vi "Fpga_v5.vi"() -> ()   [LabVIEW 2015]
uses:
  <vilib>/rvi/Emulation/niFpgaGetClockAttributes.vi
  <vilib>/rvi/Emulation/niFpgaSctlEmulationGetInTimedLoop.vi
  <vilib>/rvi/Emulation/niFpgaEmulationReportErrorSimple.vi
  <vilib>/rvi/eio/common/nirviEmuTemplateMethod_errors.vi
  <vilib>/rvi/Emulation/niFpgaCriticalErrorInLSC.vi
  <vilib>/rvi/interface/RandomDataEmulation/niFpgaRandomDataHandleErrors.vi
  <vilib>/eio/EIONode/EIONode.xnode
  <vilib>/rvi/DataTransferAndStorage/Container/XNode/niFpgaContainer.xnode
  <vilib>/rvi/interface/RandomDataEmulation/nirviRandomDataFpgaReadWriteTemplate.vi
panel:
  out "x-y 4":u32
  out "Mod2/DIO6_B 2":bool
  out "x-y":u32
  in  "Data write ON/OFF":bool
  out "Mod2/DIO6_B":bool
  out "Timed Out?":bool
  out "x-y 3":u32
  in  "stop":bool
  in  "Mod4/AO0 2":i16
  out "Mod3/AI0 2":fxp<+/-,16,5>
  out "Boolean 2":bool
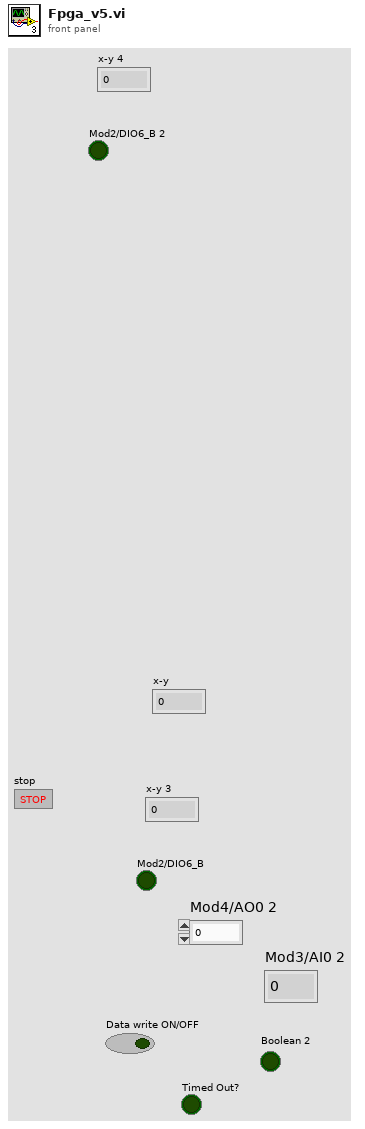
[diagram p1: front panel]
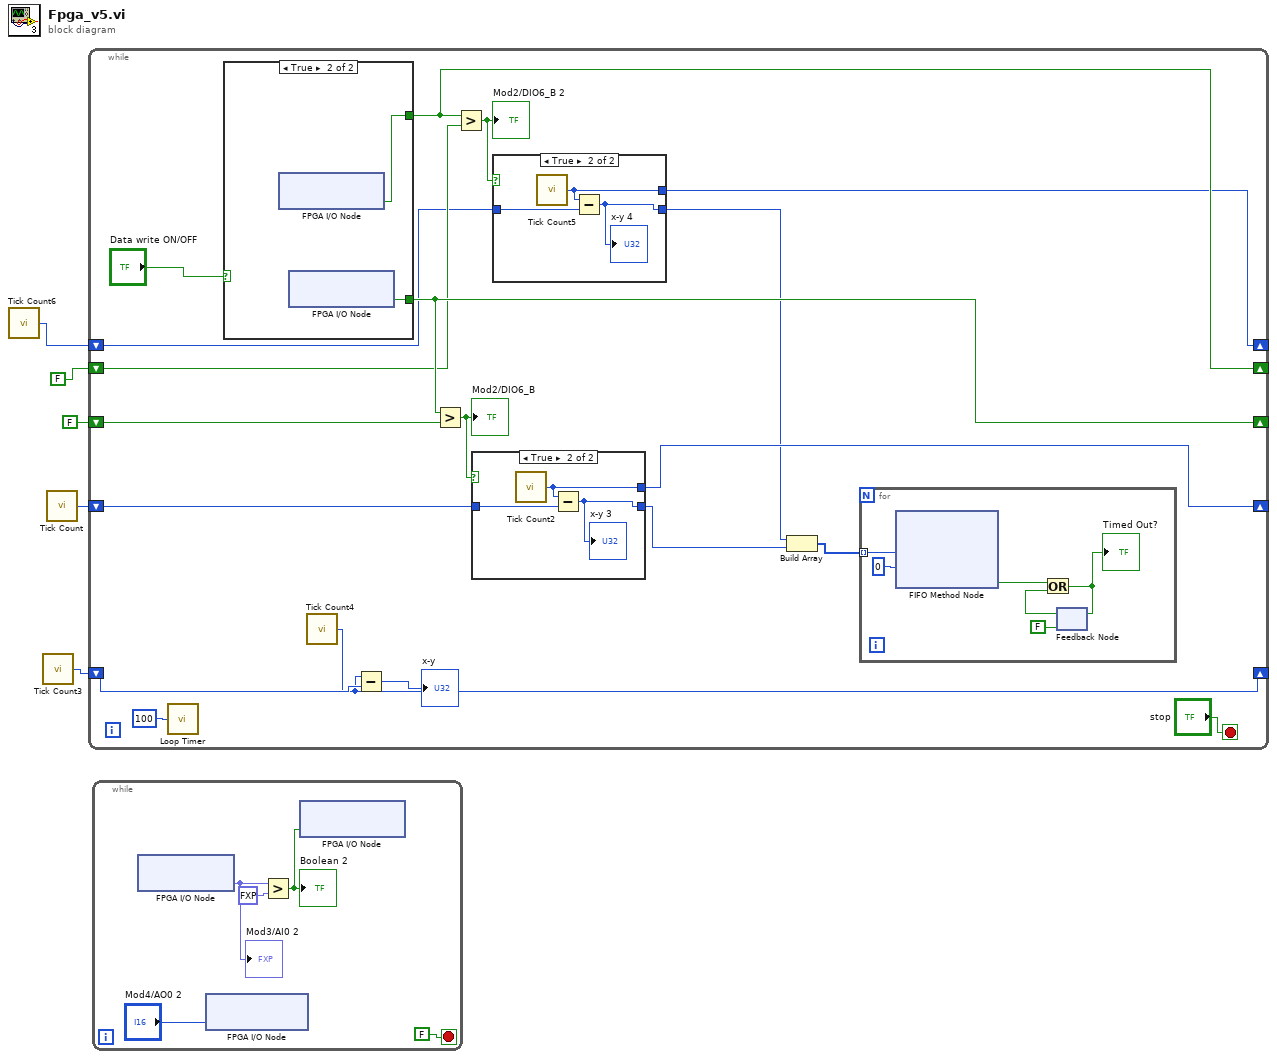
[diagram p0: block diagram]
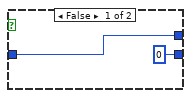
[diagram p2: hidden frame]
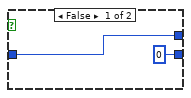
[diagram p3: hidden frame]
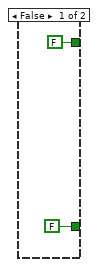
[diagram p4: hidden frame]
diagram:
  n1 = call "Tick Count6"() -> ("Tick Count(Ticks)"=w1:u32)
  n2 = call "Tick Count3"() -> ("Tick Count(Ticks)"=w3:u32)
  n3 = call "Tick Count"() -> ("Tick Count(Ticks)"=w5:u32)
  n4 = while {
    shift-right: [w21] -> _
    shift-left: w5 -> [w22]
    shift-right: [w23] -> _
    shift-left: FALSE -> [w24]
    shift-right: [w15] -> _
    shift-left: w3 -> [w16]
    shift-right: [w12] -> _
    shift-left: FALSE -> [w11]
    shift-right: [w9] -> _
    shift-left: w1 -> [w10]
    stop <- "stop" stop-if-true
    n5 = call "Loop Timer"("Count(uSec)"=u32 100) -> ()  [unwired: 1 out]
    n6 = case shown="True" "Data write ON/OFF" {
      tunnel: [FALSE ("Mod2/DIO6") w44] -> w23
      tunnel: [FALSE ("Mod2/DIO7") w43] -> w12
      frame False {
      }
      frame True {
        n7 = xnode "FPGA I/O Node"() -> ("Mod2/DIO7"=w43:bool)  [unwired: 1 in, 1 out]
        n8 = xnode "FPGA I/O Node"() -> ("Mod2/DIO6"=w44:bool)  [unwired: 1 in, 1 out]
      }
    }
    n9 = call "Tick Count4"() -> ("Tick Count(Ticks)"=w15:u32)
    n10 = Subtract(x=w15, y=w16) -> (x-y=→"x-y":u32)
    n11 = Greater?(x=w23, y=w24) -> (0:w20:bool)
    "Mod2/DIO6_B" <- w20
    n12 = Greater?(x=w12, y=w11) -> (0:w13:bool)
    "Mod2/DIO6_B 2" <- w13
    n13 = case shown="True" w20 {
      tunnel: w22 -> [w37 w40]
      tunnel: [w37 w38] -> w21
      tunnel: [u32 0 w39] -> w8
      frame False {
      }
      frame True {
        n14 = call "Tick Count2"() -> ("Tick Count(Ticks)"=w38:u32)
        n15 = Subtract(x=w38, y=w40) -> (x-y=w39:u32)
        "x-y 3" <- w39
      }
    }
    n16 = case shown="True" w13 {
      tunnel: w10 -> [w32 w35]
      tunnel: [w32 w33] -> w9
      tunnel: [u32 0 w34] -> w7
      frame False {
      }
      frame True {
        n17 = call "Tick Count5"() -> ("Tick Count(Ticks)"=w33:u32)
        n18 = Subtract(x=w33, y=w35) -> (x-y=w34:u32)
        "x-y 4" <- w34
      }
    }
    n19 = Build Array(w7, w8) -> (w6:u32[])
    n20 = for {
      tunnel: w6 -> [w25] mode=indexing
      n21 = xnode ("FIFO Method Node")("Element"=w25, "Timeout"=0) -> ("Timed Out?"=w27:bool)  [unwired: 1 in, 1 out]
      n22 = feedback #1(FALSE) -> (w28:bool)
      n23 = Or(x=w27, y=w28) -> (x .or. y?=w30:bool)
      "Timed Out?" <- w30
      n24 = feedback-in #1(w30) -> ()
    }
  }
  n25 = while {
    stop <- FALSE stop-if-true
    n26 = xnode "FPGA I/O Node"() -> ("Mod3/AI0"=w47:fxp<+/-,16,5>)  [unwired: 1 in, 1 out]
    "Mod3/AI0 2" <- w47
    n27 = xnode "FPGA I/O Node"("Mod4/AO0"="Mod4/AO0 2") -> ()  [unwired: 1 in, 1 out]
    n28 = Greater?(x=w47, y=fxp<+/-,16,5> 2.0) -> (0:w49:bool)
    "Boolean 2" <- w49
    n29 = xnode "FPGA I/O Node"("Mod2/DIO0"=w49) -> ()  [unwired: 1 in, 1 out]
  }
